vi "Camera.vi"(7 "Machine Vision":T1, 8 "error in (no error)":errorcluster, 10 "Stop":bool, 11 "Camera in":refnum<class "Camera.lvclass">) -> (0 "error out":errorcluster, 1 "Camera":dbl[](array[numeric]), 2 "Image":T3(plugin-control), 3 "Camera out":refnum<class "Camera.lvclass">, 5 "Focus output":dbl)   [LabVIEW 2016, in "Camera.lvclass"]
uses:
  Camera.lvclass
  Machine Vision.ctl
  <vilib>/Analysis/coordinate.llb/2D Cartesian Coordinate Rotation (Scalar).vi
  <vilib>/Analysis/NI_AALPro.lvlib
panel:
  out "Fitted Circle (Find Circular Edge 1)":T2 {"Average SNR (dB)" format="%.2f"; "Average Strength" format="%.2f"; "Roundness (Real-World)" format="%.2f"; "Radius (Real-World)" format="%.2f"; "Center (Real-World)"."Y" format="%.2f"; "Center (Real-World)"."X" format="%.2f"; "Radius (Pixels)" format="%.2f"; "Center (Pixels)"."Y" format="%.2f"; "Center (Pixels)"."X" format="%.2f"}
  out "subarray 2":sgl[](array[numeric])
  out "subarray":sgl[](array[numeric])
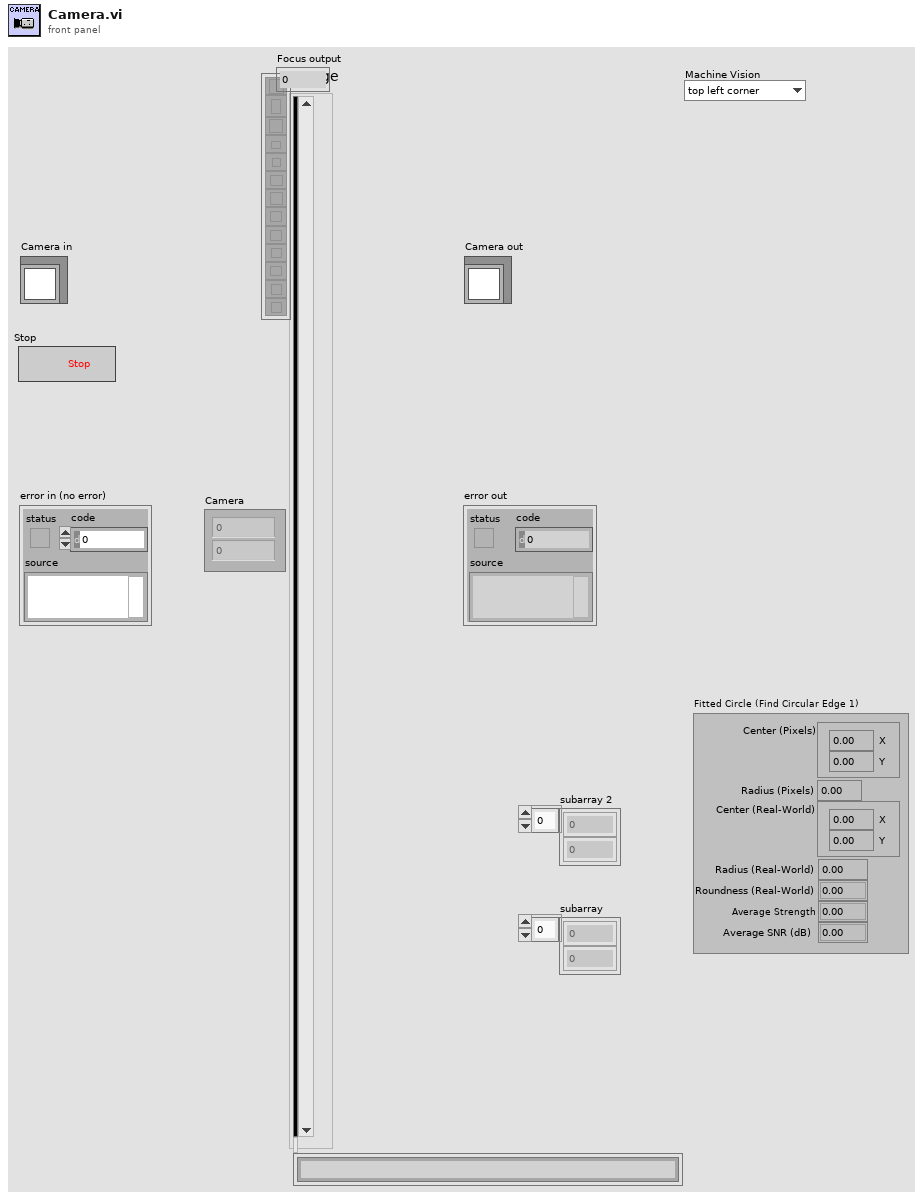
[diagram p1: front panel]
types:
  T1 = typedef "Camera.lvclass/Machine Vision.ctl" = enum16{"top left corner", "top right corner", "bottom left corner", "bottom right corner", "bottom left chip", "top right chip", "None", "tracker fiducial", "chip cross 2", "chip cross", "Focus", "INTT HDI Mark", "INTT Sensor Cross", "INTT Chip Corner", "HPK Silicon", "HPK Silicon square", "8inch PCB Pad ", "8inch PCB Pad2", "Circle", "tpcb_hole"}
  T2 = cluster{"Center (Pixels)":cluster{"X":sgl, "Y":sgl}, "Radius (Pixels)":dbl, "Center (Real-World)":cluster{"X":sgl, "Y":sgl}, "Radius (Real-World)":dbl, "Roundness (Real-World)":dbl, "Average Strength":dbl, "Average SNR (dB)":dbl}
  T3 = typedef "IMAQ Image.ctl" = refnum<image>
  T4 = typedef "IMAQ GM Match Report.ctl" = cluster{"Position":cluster{"x":sgl, "y":sgl}, "Angle":sgl, "Scale":sgl, "Score":sgl, "Bounding Box":cluster{"x":sgl, "y":sgl}[], "Contrast Reversed":bool, "Occlusion %":sgl, "Template Target Curve Score":sgl, "Target Template Curve Score":sgl, "Correlation Score":sgl}
  T5 = cluster{"Position":cluster{"x":sgl, "y":sgl}, "Angle":sgl, "Scale":sgl, "Score":sgl, "Bounding Box":cluster{"x":sgl, "y":sgl}[]}[]
  T6 = cluster{"Position":cluster{"x":sgl, "y":sgl}, "Angle":sgl, "Scale":sgl, "Score":sgl, "Bounding Box":cluster{"x":sgl, "y":sgl}[]}
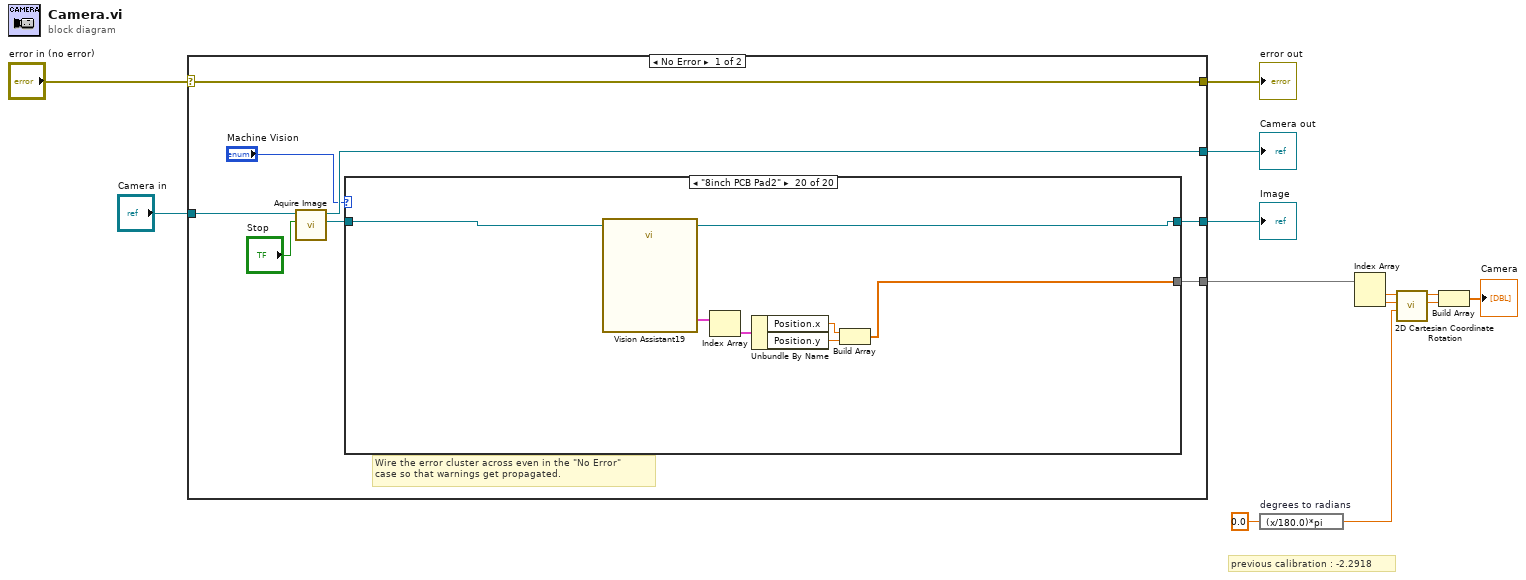
[diagram p0: block diagram]
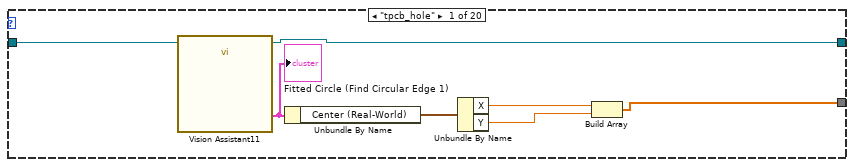
[diagram p2: hidden frame]
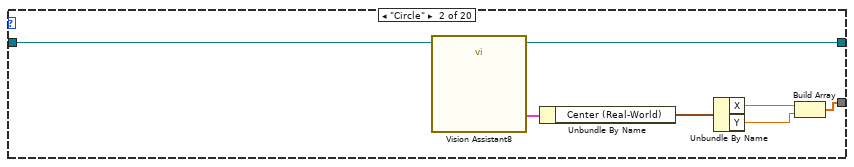
[diagram p3: hidden frame]
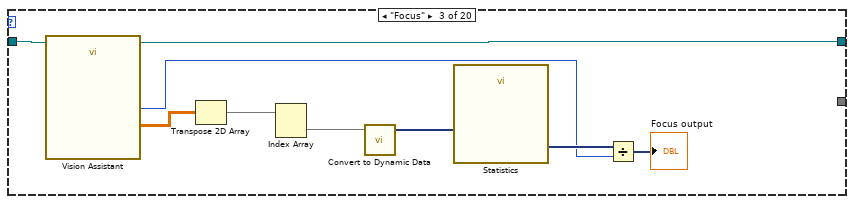
[diagram p4: hidden frame]
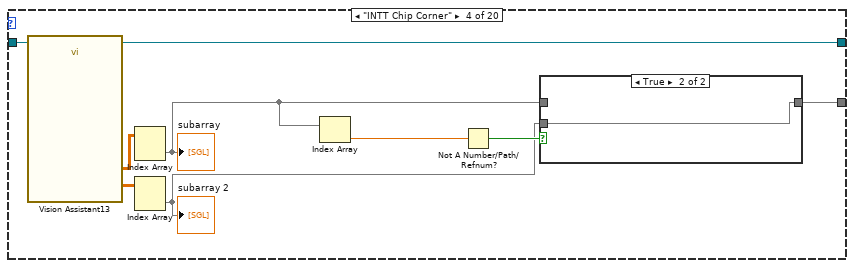
[diagram p5: hidden frame]
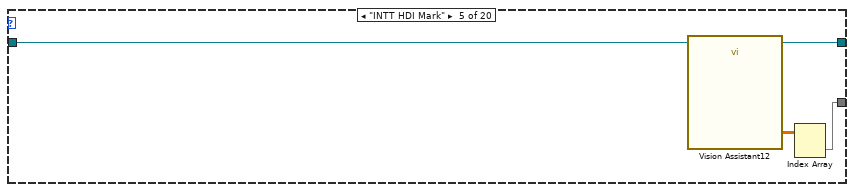
[diagram p7: hidden frame]
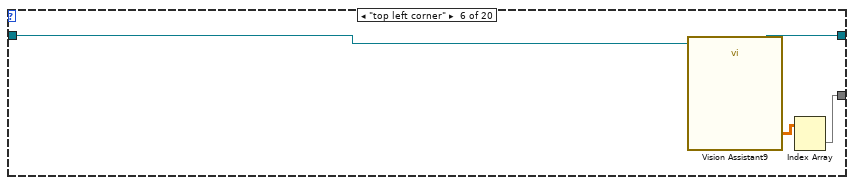
[diagram p8: hidden frame]
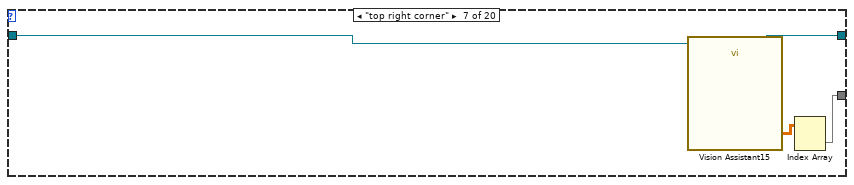
[diagram p9: hidden frame]
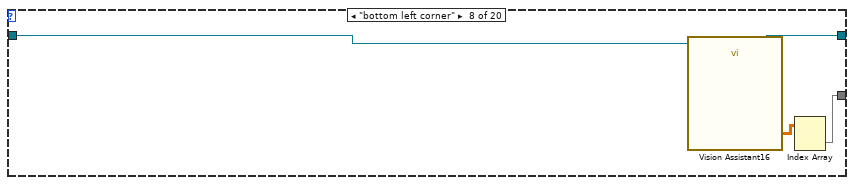
[diagram p10: hidden frame]
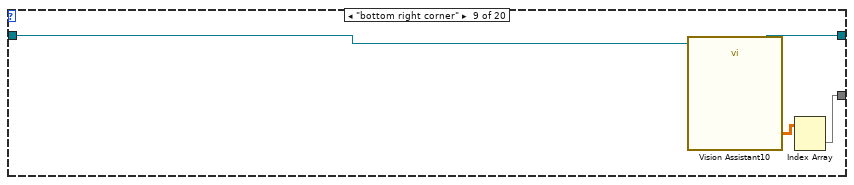
[diagram p11: hidden frame]
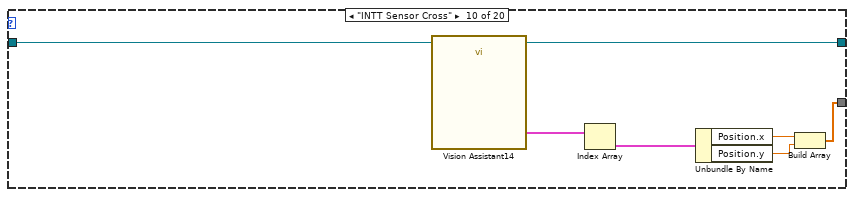
[diagram p12: hidden frame]
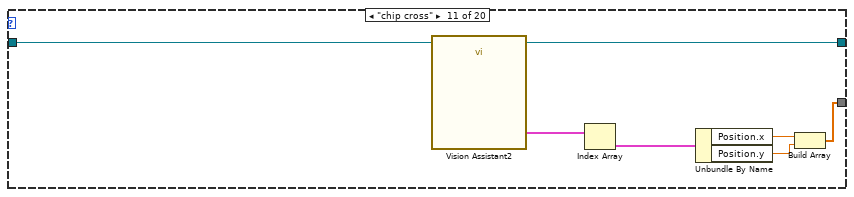
[diagram p13: hidden frame]
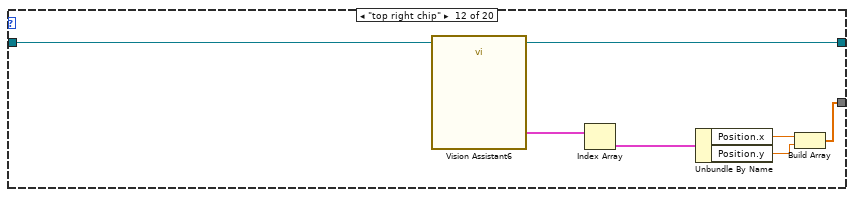
[diagram p14: hidden frame]
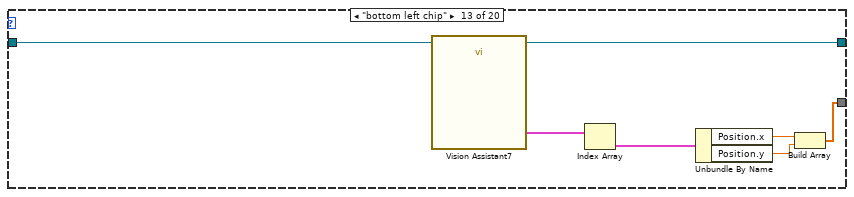
[diagram p15: hidden frame]
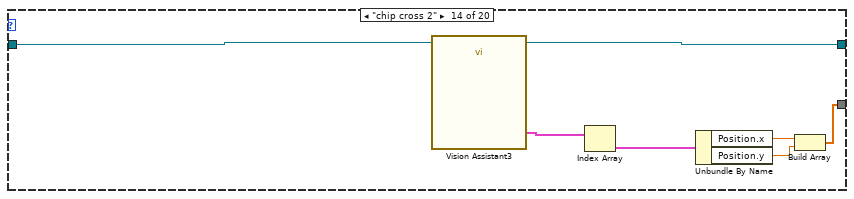
[diagram p16: hidden frame]
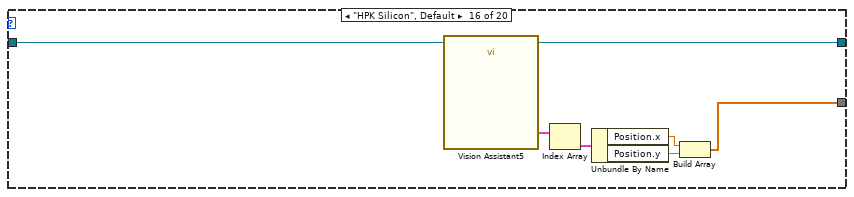
[diagram p18: hidden frame]
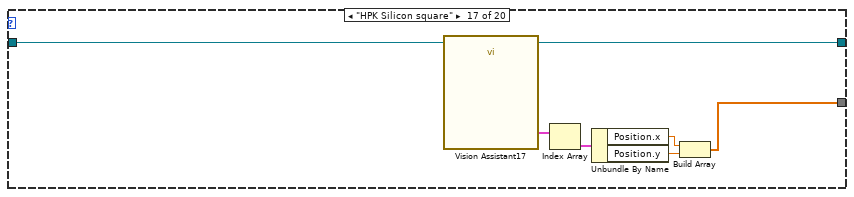
[diagram p19: hidden frame]
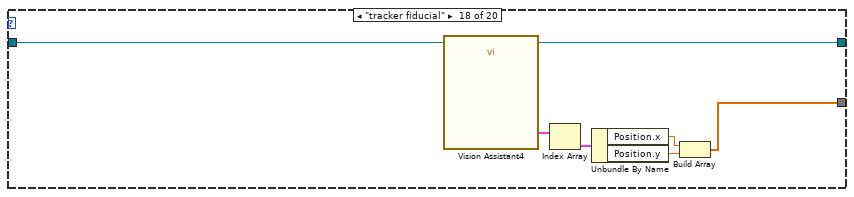
[diagram p20: hidden frame]
diagram:
  # "previous calibration : -2.2918"
  n1 = case shown="No Error" "error in (no error)" {
    selector: "error in (no error)" -> [w21 w148]
    tunnel: [w21 w148] -> w12
    tunnel: [w18 w147] -> w11
    tunnel: "Camera in" -> [w19 w147]
    tunnel: [w17 _] -> w6
    tunnel: [w16 _] -> w9
    frame No Error {
      # "Wire the error cluster across even in the \"No Error\"\ncase so that warnings get propagated."
      n2 = call-dynamic "Aquire Image.vi"("Stop"="Stop", "Camera in"=w19) -> ("Image Out"=w15:T3, "Camera out"=w18:refnum<class "Camera.lvclass">)  [unwired: 7 in, 1 out]
      n3 = case shown="\"8inch PCB Pad2\"" "Machine Vision" {
        tunnel: [w22 w29 _ w45 w57 w61 w65 w69 w73 w78 w85 w92 w99 w106 _ w112 w119 w126 w134 w140] -> w17
        tunnel: [w23 w34 w43 w48 w58 w62 w66 w70 w74 w77 w84 w91 w98 w105 w111 w118 w125 w132 w135 w141] -> w16
        tunnel: w15 -> [w25 w35 w44 w47 w59 w63 w67 w71 w75 w76 w83 w90 w97 w104 w111 w117 w124 w131 w133 w142]
        frame "tpcb_hole" {
          n4 = call "Vision Assistant11"("Image In"=w25) -> ("Image Out"=w23:T3, "Fitted Circle (Find Circular Edge 1)"=w24:T2)  [unwired: 24 in, 1 out]
          "Fitted Circle (Find Circular Edge 1)" <- w24
          n5 = Unbundle By Name(w24) -> ("Center (Real-World)"=w28:cluster{"X":sgl, "Y":sgl})
          n6 = Unbundle By Name(w28) -> ("X"=w27:sgl, "Y"=w26:sgl)
          n7 = Build Array(w27, w26) -> (w22:sgl[])
        }
        frame "Circle" {
          n8 = call "Vision Assistant8"("Image In"=w35) -> ("Image Out"=w34:T3, "Fitted Circle (Find Circular Edge 1)"=w30:T2)  [unwired: 24 in, 1 out]
          n9 = Unbundle By Name(w30) -> ("Center (Real-World)"=w33:cluster{"X":sgl, "Y":sgl})
          n10 = Unbundle By Name(w33) -> ("X"=w32:sgl, "Y"=w31:sgl)
          n11 = Build Array(w32, w31) -> (w29:sgl[])
        }
        frame "Focus" {
          n12 = call "Vision Assistant"("Image In"=w44) -> ("Image Out"=w43:T3, "Number of Particles (Particle Analysis 1)"=w37:i32, "Particle Measurements (Pixels) (Particle Analysis 1)"=w36:dbl[][])  [unwired: 22 in, 2 out]
          n13 = Transpose 2D Array(2D array=w36) -> (transposed array=w42:dbl[][])
          n14 = Index Array(array=w42) -> (element=w41:dbl[])  [unwired: 2 in]
          n15 = call "Convert to Dynamic Data"("Array"=w41) -> ("Dynamic Data Type"=w40:dynamicdata)  [unwired: 3 in]
          n16 = call "Statistics"("Signals"=w40) -> ("Summation"=w39:dynamicdata)  [unwired: 25 in, 1 out]
          n17 = Divide(x=w39, y=w37) -> (x/y=→"Focus output":dynamicdata)
        }
        frame "INTT Chip Corner" {
          n18 = call "Vision Assistant13"("Image In"=w47) -> ("Image Out"=w48:T3, "Calibrated Results (Caliper 1)"=w53:sgl[][], "Calibrated Results (Caliper 2)"=w50:sgl[][])  [unwired: 17 in, 7 out]
          n19 = Index Array(array=w53) -> (element=w46:sgl[])  [unwired: 2 in]
          "subarray" <- w46
          n20 = Index Array(array=w50) -> (element=w49:sgl[])  [unwired: 2 in]
          "subarray 2" <- w49
          n21 = Index Array(array=w46) -> (element=w52:sgl)  [unwired: 1 in]
          n22 = Not A Number/Path/Refnum?(number/path/refnum=w52) -> (NaN/Path/Refnum?=w51:bool)
          n23 = case shown="True" w51 {
            tunnel: w46 -> [w54 _]
            tunnel: w49 -> [_ w55]
            tunnel: [w54 w55] -> w45
            frame False {
            }
            frame True {
            }
          }
        }
        frame "INTT HDI Mark" {
          n24 = call "Vision Assistant12"("Image In"=w59) -> ("Image Out"=w58:T3, "Calibrated Results (Caliper 5)"=w56:sgl[][])  [unwired: 21 in, 4 out]
          n25 = Index Array(array=w56) -> (element=w57:sgl[])  [unwired: 2 in]
        }
        frame "top left corner" {
          n26 = call "Vision Assistant9"("Image In"=w63) -> ("Image Out"=w62:T3, "Calibrated Results (Caliper 6)"=w60:sgl[][])  [unwired: 23 in, 2 out]
          n27 = Index Array(array=w60) -> (element=w61:sgl[])  [unwired: 2 in]
        }
        frame "top right corner" {
          n28 = call "Vision Assistant15"("Image In"=w67) -> ("Image Out"=w66:T3, "Calibrated Results (Caliper 6)"=w64:sgl[][])  [unwired: 23 in, 2 out]
          n29 = Index Array(array=w64) -> (element=w65:sgl[])  [unwired: 2 in]
        }
        frame "bottom left corner" {
          n30 = call "Vision Assistant16"("Image In"=w71) -> ("Image Out"=w70:T3, "Calibrated Results (Caliper 6)"=w68:sgl[][])  [unwired: 23 in, 2 out]
          n31 = Index Array(array=w68) -> (element=w69:sgl[])  [unwired: 2 in]
        }
        frame "bottom right corner" {
          n32 = call "Vision Assistant10"("Image In"=w75) -> ("Image Out"=w74:T3, "Calibrated Results (Caliper 6)"=w72:sgl[][])  [unwired: 23 in, 2 out]
          n33 = Index Array(array=w72) -> (element=w73:sgl[])  [unwired: 2 in]
        }
        frame "INTT Sensor Cross" {
          n34 = call "Vision Assistant14"("Image In"=w76) -> ("Image Out"=w77:T3, "Calibrated Matches (Geometric Matching 1)"=w82:T4[])  [unwired: 23 in, 2 out]
          n35 = Index Array(array=w82) -> (element=w81:T4)  [unwired: 1 in]
          n36 = Unbundle By Name(w81) -> ("Position.x"=w80:sgl, "Position.y"=w79:sgl)
          n37 = Build Array(w80, w79) -> (w78:sgl[])
        }
        frame "chip cross" {
          n38 = call "Vision Assistant2"("Image In"=w83) -> ("Image Out"=w84:T3, "Calibrated Matches (Geometric Matching 1)"=w89:T4[])  [unwired: 23 in, 2 out]
          n39 = Index Array(array=w89) -> (element=w88:T4)  [unwired: 1 in]
          n40 = Unbundle By Name(w88) -> ("Position.x"=w87:sgl, "Position.y"=w86:sgl)
          n41 = Build Array(w87, w86) -> (w85:sgl[])
        }
        frame "top right chip" {
          n42 = call "Vision Assistant6"("Image In"=w90) -> ("Image Out"=w91:T3, "Calibrated Matches (Geometric Matching 1)"=w96:T4[])  [unwired: 23 in, 2 out]
          n43 = Index Array(array=w96) -> (element=w95:T4)  [unwired: 1 in]
          n44 = Unbundle By Name(w95) -> ("Position.x"=w94:sgl, "Position.y"=w93:sgl)
          n45 = Build Array(w94, w93) -> (w92:sgl[])
        }
        frame "bottom left chip" {
          n46 = call "Vision Assistant7"("Image In"=w97) -> ("Image Out"=w98:T3, "Calibrated Matches (Geometric Matching 1)"=w103:T4[])  [unwired: 23 in, 2 out]
          n47 = Index Array(array=w103) -> (element=w102:T4)  [unwired: 1 in]
          n48 = Unbundle By Name(w102) -> ("Position.x"=w101:sgl, "Position.y"=w100:sgl)
          n49 = Build Array(w101, w100) -> (w99:sgl[])
        }
        frame "chip cross 2" {
          n50 = call "Vision Assistant3"("Image In"=w104) -> ("Image Out"=w105:T3, "Calibrated Matches (Geometric Matching 1)"=w110:T4[])  [unwired: 23 in, 2 out]
          n51 = Index Array(array=w110) -> (element=w109:T4)  [unwired: 1 in]
          n52 = Unbundle By Name(w109) -> ("Position.x"=w108:sgl, "Position.y"=w107:sgl)
          n53 = Build Array(w108, w107) -> (w106:sgl[])
        }
        frame "None" {
        }
        frame "HPK Silicon", Default {
          n54 = call "Vision Assistant5"("Image In"=w117) -> ("Image Out"=w118:T3, "Calibrated Matches (Geometric Matching 1)"=w113:T4[])  [unwired: 23 in, 2 out]
          n55 = Index Array(array=w113) -> (element=w116:T4)  [unwired: 1 in]
          n56 = Unbundle By Name(w116) -> ("Position.x"=w115:sgl, "Position.y"=w114:sgl)
          n57 = Build Array(w115, w114) -> (w112:sgl[])
        }
        frame "HPK Silicon square" {
          n58 = call "Vision Assistant17"("Image In"=w124) -> ("Image Out"=w125:T3, "Calibrated Matches (Pattern Matching 1)"=w120:T5)  [unwired: 23 in, 2 out]
          n59 = Index Array(array=w120) -> (element=w123:T6)  [unwired: 1 in]
          n60 = Unbundle By Name(w123) -> ("Position.x"=w122:sgl, "Position.y"=w121:sgl)
          n61 = Build Array(w122, w121) -> (w119:sgl[])
        }
        frame "tracker fiducial" {
          n62 = call "Vision Assistant4"("Image In"=w131) -> ("Image Out"=w132:T3, "Calibrated Matches (Geometric Matching 1)"=w127:T4[])  [unwired: 23 in, 2 out]
          n63 = Index Array(array=w127) -> (element=w130:T4)  [unwired: 1 in]
          n64 = Unbundle By Name(w130) -> ("Position.x"=w129:sgl, "Position.y"=w128:sgl)
          n65 = Build Array(w129, w128) -> (w126:sgl[])
        }
        frame "8inch PCB Pad " {
          n66 = call "Vision Assistant18"("Image In"=w133) -> ("Image Out"=w135:T3, "Calibrated Matches (Pattern Matching 1)"=w139:T5)  [unwired: 23 in, 2 out]
          n67 = Index Array(array=w139) -> (element=w136:T6)  [unwired: 1 in]
          n68 = Unbundle By Name(w136) -> ("Position.x"=w137:sgl, "Position.y"=w138:sgl)
          n69 = Build Array(w137, w138) -> (w134:sgl[])
        }
        frame "8inch PCB Pad2" {
          n70 = call "Vision Assistant19"("Image In"=w142) -> ("Image Out"=w141:T3, "Calibrated Matches (Pattern Matching 1)"=w143:T5)  [unwired: 23 in, 2 out]
          n71 = Index Array(array=w143) -> (element=w146:T6)  [unwired: 1 in]
          n72 = Unbundle By Name(w146) -> ("Position.x"=w145:sgl, "Position.y"=w144:sgl)
          n73 = Build Array(w145, w144) -> (w140:sgl[])
        }
      }
    }
    frame Error {
    }
  }
  "error out" <- w12
  "Camera out" <- w11
  "Image" <- w9
  n74 = expression code="(x/180.0)*pi" "degrees to radians"(0.0) -> (w3:dbl)
  n75 = Index Array(array=w6) -> (element #1=w5:sgl, element #2=w4:sgl)  [unwired: 2 in]
  n76 = call-poly <vilib>:"2D Cartesian Coordinate Rotation.vi"("theta"=w3, "y"=w4, "x"=w5) -> ("y out"=w1:dbl, "x out"=w7:dbl)  [unwired: 6 in, 1 out]
  n77 = Build Array(w7, w1) -> (→"Camera":dbl[])
